vi "Native POST Multipart File Upload Example.vi"() -> ()   [LabVIEW 2017]
uses:
  <vilib>/httpClient/MultipartData.ctl
  <vilib>/httpClient/LabVIEWHTTPClient.lvlib
panel:
  out "body":string
  out "headers":string
  in  "Authentication":cluster{"Username":string, "Password":string}
  out "error out":errorcluster
  in  "FIlepath":path=path "D:/upwork/Labview-REST-API/labview-source/payload.png"
  in  "API Endpoint Url":string="https://api.dev.enlil.io/api/v1/attachments/external/upload"
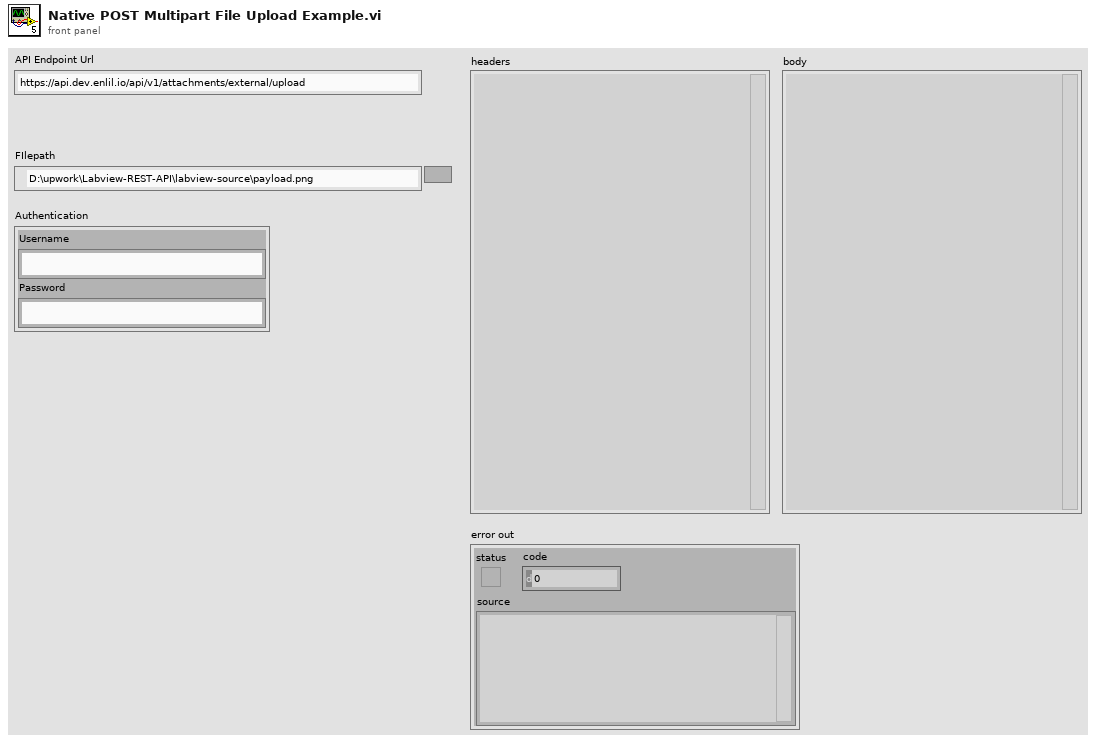
[diagram p1: front panel]
types:
  T1 = typedef "LabVIEWHTTPClient.lvlib/MultipartData.ctl" = cluster{"Name":string, "Value":string, "File":path, "Filename":string, "MIME type":string}
  T2 = typedef "LabVIEWHTTPClient.lvlib/ClientHandle.ctl" = refnum<k1>
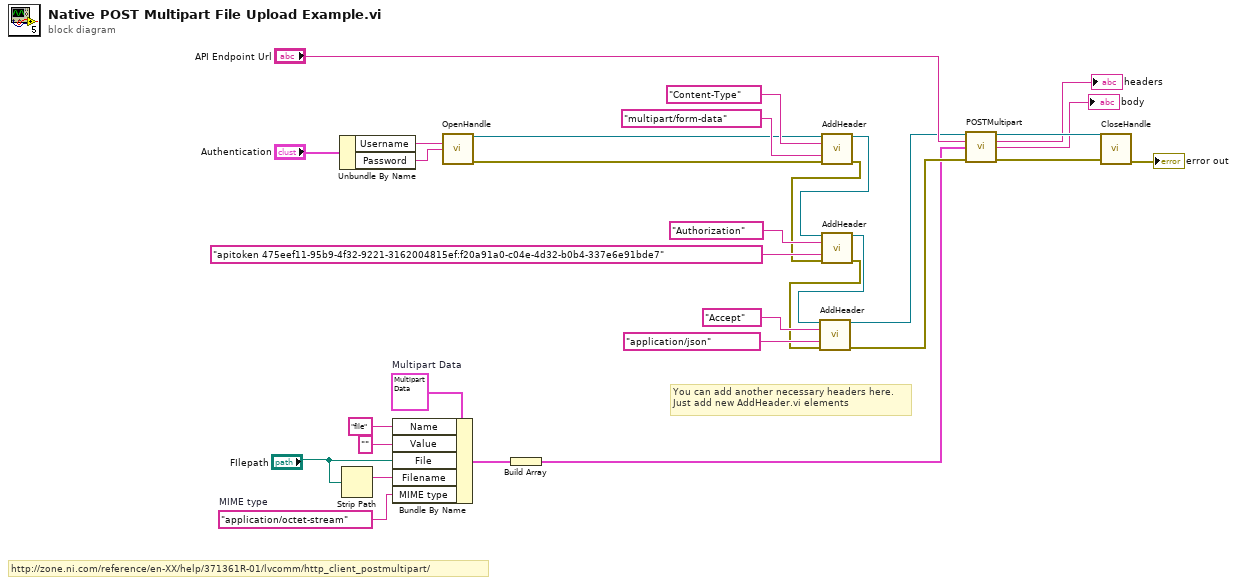
[diagram p0: block diagram]
diagram:
  w18 = "application/octet-stream"  # MIME type
  w22 = T1 {"Name"="", "Value"="", "File"=path "", "Filename"="", "MIME type"="application/octet-stream"}  # Multipart Data
  # "You can add another necessary headers here.\nJust add new AddHeader.vi elements"
  # "http://zone.ni.com/reference/en-XX/help/371361R-01/lvcomm/http_client_postmultipart/"
  n1 = Unbundle By Name("Authentication") -> ("Username"=w30:string, "Password"=w29:string)
  n2 = Strip Path(path="FIlepath") -> (name=w19:string)  [unwired: 1 out]
  n3 = Bundle By Name(cluster=w22, "Name"="file", "Value"="", "File"="FIlepath", "Filename"=w19, "MIME type"=w18) -> (w17:T1)
  n4 = call <vilib>:"OpenHandle.vi"("username"=w30, "password"=w29) -> ("client handle out"=w5:T2, "error out"=w4:errorcluster)  [unwired: 12 in]
  n5 = Build Array(w17) -> (w1:T1[])
  n6 = call <vilib>:"AddHeader.vi"("client handle"=w5, "header"="Content-Type", "value"="multipart/form-data", "error in (no error)"=w4) -> ("client handle out"=w9:T2, "error out"=w8:errorcluster)  [unwired: 10 in]
  n7 = call <vilib>:"AddHeader.vi"("client handle"=w9, "header"="Authorization", "value"="apitoken 475eef11-95b9-4f32-9221-3162004815ef:f20a91a0-c04e-4d32-b0b4-337e6e91bde7", "error in (no error)"=w8) -> ("client handle out"=w7:T2, "error out"=w6:errorcluster)  [unwired: 10 in]
  n8 = call <vilib>:"AddHeader.vi"("client handle"=w7, "header"="Accept", "value"="application/json", "error in (no error)"=w6) -> ("client handle out"=w3:T2, "error out"=w2:errorcluster)  [unwired: 10 in]
  n9 = call <vilib>:"POSTMultipart.vi"("client handle"=w3, "url"="API Endpoint Url", "data"=w1, "error in (no error)"=w2) -> ("client handle out"=w27:T2, "headers"=→"headers":string, "body"=→"body":string, "error out"=w26:errorcluster)  [unwired: 8 in]
  n10 = call <vilib>:"CloseHandle.vi"("client handle"=w27, "error in (no error)"=w26) -> ("error out"=→"error out":errorcluster)  [unwired: 13 in]
